vi "中英文.vi"(0 "中英文":string="English") -> ()   [LabVIEW 2018]
panel:
  out "all rows":string[](array[string])
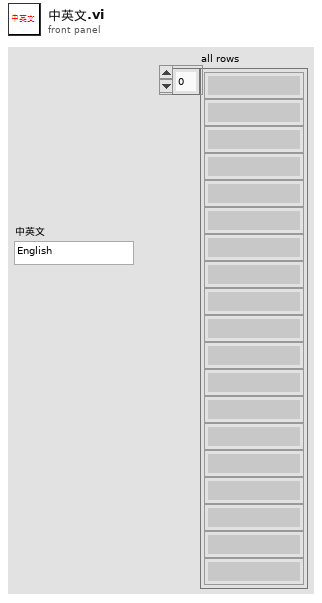
[diagram p1: front panel]
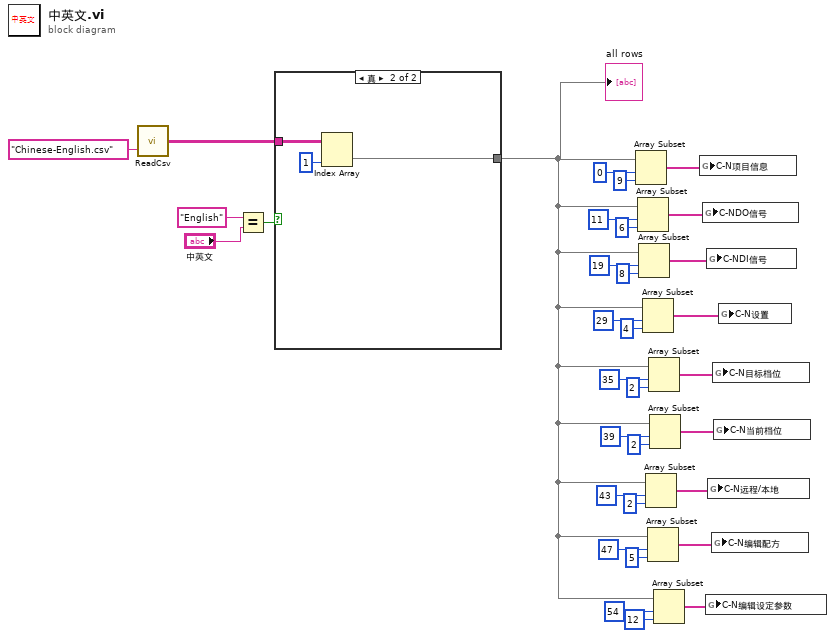
[diagram p0: block diagram]
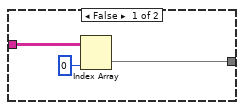
[diagram p2: hidden frame]
diagram:
  n1 = call "ReadCsv.vi"("相对路径"="Chinese-English.csv") -> ("all rows"=w29:string[][])  [unwired: 1 in]
  n2 = Equal?(x="English", y="中英文") -> (x = y?=w32:bool)
  n3 = case shown="真" w32 {
    tunnel: w29 -> [w35 w39]
    tunnel: [w34 w37] -> w1
    frame False {
      n4 = Index Array(array=w35, index (col)=0 ("禁用的索引 (列)")) -> (element=w34:string[])  [unwired: 1 in]
    }
    frame True {
      n5 = Index Array(array=w39, index (col)=1 ("禁用的索引 (列)")) -> (element=w37:string[])  [unwired: 1 in]
    }
  }
  "all rows" <- w1
  n6 = Array Subset(array=w1, index=0 ("索引"), length=9 ("长度")) -> (w28:string[])
  n7 = Array Subset(array=w1, index=11 ("索引"), length=6 ("长度")) -> (w23:string[])
  n8 = Array Subset(array=w1, index=19 ("索引"), length=8 ("长度")) -> (w22:string[])
  n9 = Array Subset(array=w1, index=29 ("索引"), length=4 ("长度")) -> (w17:string[])
  n10 = Array Subset(array=w1, index=43 ("索引"), length=2 ("长度")) -> (w10:string[])
  n11 = Array Subset(array=w1, index=47 ("索引"), length=5 ("长度")) -> (w5:string[])
  n12 = Array Subset(array=w1, index=35 ("索引"), length=2 ("长度")) -> (w16:string[])
  n13 = Array Subset(array=w1, index=39 ("索引"), length=2 ("长度")) -> (w11:string[])
  n14 = Array Subset(array=w1, index=54 ("索引"), length=12 ("长度")) -> (w4:string[])
  n15 = global write "全局 1.vi" "C-N项目信息"(w28) -> ()
  n16 = global write "全局 1.vi" "C-NDO信号"(w23) -> ()
  n17 = global write "全局 1.vi" "C-N编辑设定参数"(w4) -> ()
  n18 = global write "全局 1.vi" "C-NDI信号"(w22) -> ()
  n19 = global write "全局 1.vi" "C-N远程/本地"(w10) -> ()
  n20 = global write "全局 1.vi" "C-N编辑配方"(w5) -> ()
  n21 = global write "全局 1.vi" "C-N目标档位"(w16) -> ()
  n22 = global write "全局 1.vi" "C-N当前档位"(w11) -> ()
  n23 = global write "全局 1.vi" "C-N设置"(w17) -> ()
